vi "Zero Adjust Pressure.vi"(8 "Error In":errorcluster, 11 "VISA resource name":refnum<visa-resource-name>) -> (0 "Error Out":errorcluster, 1 "Pressure Offset":dbl[unit], 3 "dup VISA resource name":refnum<visa-resource-name>)   [LabVIEW 2011, in "MGC647C.lvlib"]
doc: "Zero adjust pressure."
uses:
  <instrlib>/MGC647C/MGC647C.lvlib
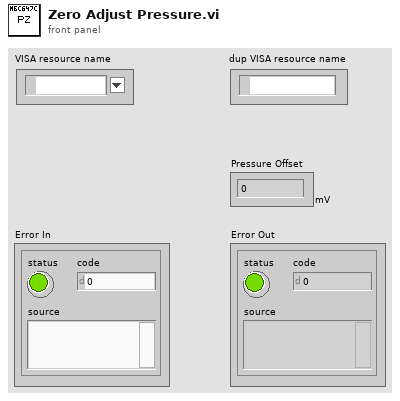
[diagram p1: front panel]
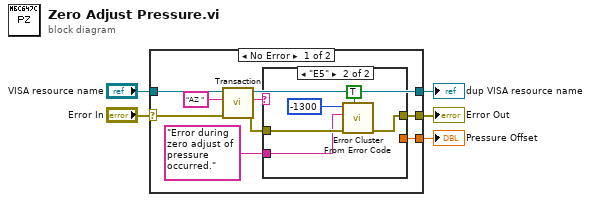
[diagram p0: block diagram]
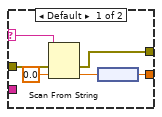
[diagram p2: hidden frame]
diagram:
  n1 = case shown="No Error" "Error In" {
    selector: "Error In" -> [w7 w27]
    tunnel: "VISA resource name" -> [w14 w26]
    tunnel: [w13 w26] -> w4
    tunnel: [w12 w27] -> w3
    tunnel: [w11 _] -> w1
    frame No Error {
      n2 = call <instrlib>:"Transaction.vi"("Error In"=w7, "Command"="AZ " ("string (\"\")"), "VISA resource name"=w14) -> ("Error Out"=w10:errorcluster, "Response"=w9:string, "dup VISA resource name"=w13:refnum<visa-resource-name>)  [unwired: 6 in]
      n3 = case shown="\"E5\"" w9 {
        selector: w9 -> [w15 _]
        tunnel: w10 -> [w20 w24]
        tunnel: [w19 w25] -> w12
        tunnel: [w16 _] -> w11
        tunnel: "Error during zero adjust of pressure occurred." ("error source (\" \")") -> [_ w22]
        frame Default {
          n4 = Scan From String(input string=w15, error in=w20, default 1=0.0 ("default value 1")) -> (error out=w19:errorcluster, output 1=w17:dbl)  [unwired: 2 in, 2 out]
          n5 = node(w17) -> (w16:dbl[unit])
        }
        frame "E5" {
          n6 = call <vilib>:"Error Cluster From Error Code.vi"("show call chain? (False)"=TRUE, "error in (no error)"=w24, "error message (\"\")"=w22, "error code (0)"=-1300 ("error code (no error:0)")) -> ("error out"=w25:errorcluster)  [unwired: 5 in]
        }
      }
    }
    frame Error {
    }
  }
  "dup VISA resource name" <- w4
  "Error Out" <- w3
  "Pressure Offset" <- w1
